vi "ManualClimb.vi"   [LabVIEW 2020]
uses:
  Robot Global Data.vi
  Swerve Global Variables.vi
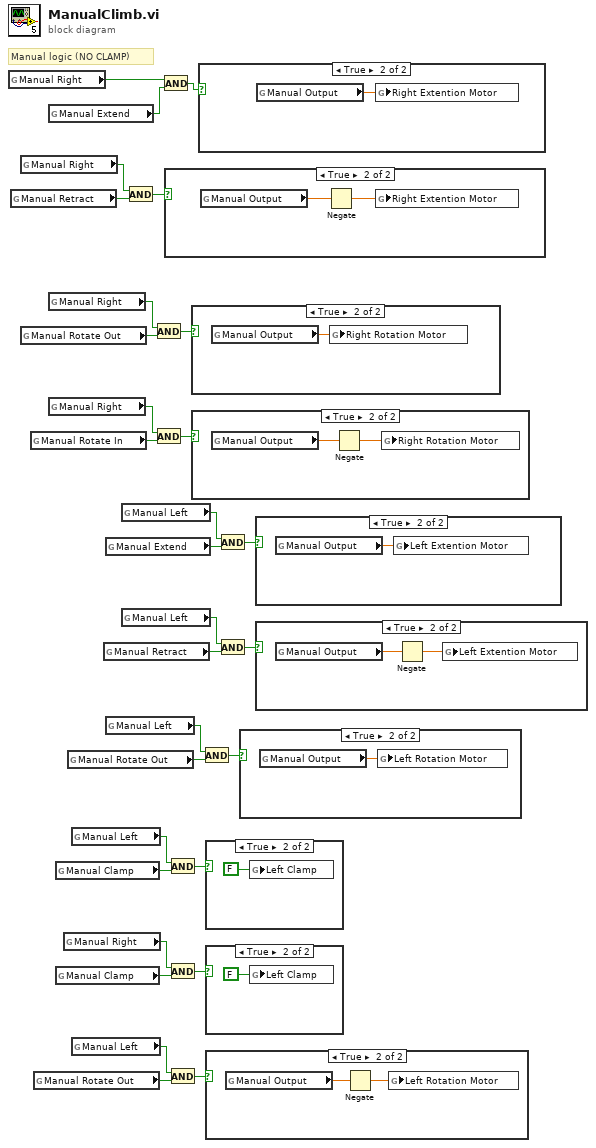
[diagram p0: block diagram]
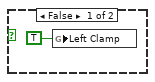
[diagram p2: hidden frame]
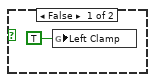
[diagram p3: hidden frame]
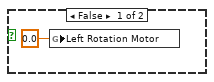
[diagram p4: hidden frame]
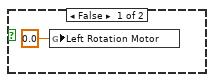
[diagram p5: hidden frame]
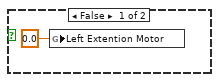
[diagram p6: hidden frame]
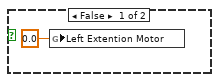
[diagram p7: hidden frame]
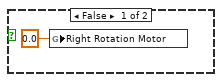
[diagram p8: hidden frame]
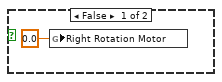
[diagram p9: hidden frame]
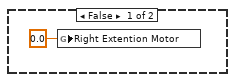
[diagram p10: hidden frame]
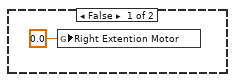
[diagram p11: hidden frame]
diagram:
  # "Manual logic (NO CLAMP)"
  n1 = global read "Robot Global Data.vi" "Manual Right"() -> (w2:bool)
  n2 = global read "Robot Global Data.vi" "Manual Retract"() -> (w5:bool)
  n3 = global read "Robot Global Data.vi" "Manual Right"() -> (w4:bool)
  n4 = global read "Robot Global Data.vi" "Manual Rotate Out"() -> (w9:bool)
  n5 = global read "Robot Global Data.vi" "Manual Rotate In"() -> (w12:bool)
  n6 = global read "Robot Global Data.vi" "Manual Rotate Out"() -> (w24:bool)
  n7 = global read "Robot Global Data.vi" "Manual Extend"() -> (w1:bool)
  n8 = global read "Robot Global Data.vi" "Manual Right"() -> (w8:bool)
  n9 = global read "Robot Global Data.vi" "Manual Right"() -> (w11:bool)
  n10 = global read "Robot Global Data.vi" "Manual Clamp"() -> (w26:bool)
  n11 = global read "Robot Global Data.vi" "Manual Clamp"() -> (w28:bool)
  n12 = global read "Robot Global Data.vi" "Manual Right"() -> (w27:bool)
  n13 = global read "Robot Global Data.vi" "Manual Rotate Out"() -> (w21:bool)
  n14 = global read "Robot Global Data.vi" "Manual Left"() -> (w25:bool)
  n15 = global read "Robot Global Data.vi" "Manual Left"() -> (w23:bool)
  n16 = global read "Robot Global Data.vi" "Manual Retract"() -> (w17:bool)
  n17 = global read "Robot Global Data.vi" "Manual Extend"() -> (w13:bool)
  n18 = global read "Robot Global Data.vi" "Manual Left"() -> (w20:bool)
  n19 = global read "Robot Global Data.vi" "Manual Left"() -> (w14:bool)
  n20 = global read "Robot Global Data.vi" "Manual Left"() -> (w16:bool)
  n21 = And(x=w4, y=w5) -> (x .and. y?=w6:bool)
  n22 = And(x=w8, y=w9) -> (x .and. y?=w7:bool)
  n23 = And(x=w11, y=w12) -> (x .and. y?=w10:bool)
  n24 = And(x=w2, y=w1) -> (x .and. y?=w3:bool)
  n25 = case shown="True" w6 {
    frame False {
      n26 = global write "Swerve Global Variables.vi" "Right Extention Motor"(0.0 ("Right Rotation Motor")) -> ()
    }
    frame True {
      n27 = global read "Swerve Global Variables.vi" "Manual Output"() -> (w33:dbl)
      n28 = Negate(x=w33) -> (-x=w32:dbl)
      n29 = global write "Swerve Global Variables.vi" "Right Extention Motor"(w32) -> ()
    }
  }
  n30 = And(x=w25, y=w26) -> (x .and. y?=w30:bool)
  n31 = And(x=w27, y=w28) -> (x .and. y?=w29:bool)
  n32 = And(x=w23, y=w24) -> (x .and. y?=w22:bool)
  n33 = case shown="True" w7 {
    frame False {
      n34 = global write "Swerve Global Variables.vi" "Right Rotation Motor"(0.0 ("Right Extention Motor")) -> ()
    }
    frame True {
      n35 = global read "Swerve Global Variables.vi" "Manual Output"() -> (w35:dbl)
      n36 = global write "Swerve Global Variables.vi" "Right Rotation Motor"(w35) -> ()
    }
  }
  n37 = case shown="True" w10 {
    frame False {
      n38 = global write "Swerve Global Variables.vi" "Right Rotation Motor"(0.0 ("Right Extention Motor")) -> ()
    }
    frame True {
      n39 = global read "Swerve Global Variables.vi" "Manual Output"() -> (w38:dbl)
      n40 = Negate(x=w38) -> (-x=w37:dbl)
      n41 = global write "Swerve Global Variables.vi" "Right Rotation Motor"(w37) -> ()
    }
  }
  n42 = case shown="True" w3 {
    frame False {
      n43 = global write "Swerve Global Variables.vi" "Right Extention Motor"(0.0 ("Right Rotation Motor")) -> ()
    }
    frame True {
      n44 = global read "Swerve Global Variables.vi" "Manual Output"() -> (w40:dbl)
      n45 = global write "Swerve Global Variables.vi" "Right Extention Motor"(w40) -> ()
    }
  }
  n46 = And(x=w20, y=w21) -> (x .and. y?=w19:bool)
  n47 = case shown="True" w30 {
    frame False {
      n48 = global write "Robot Global Data.vi" "Left Clamp"(TRUE ("Left Clamp")) -> ()
    }
    frame True {
      n49 = global write "Robot Global Data.vi" "Left Clamp"(FALSE ("Left Clamp")) -> ()
    }
  }
  n50 = case shown="True" w29 {
    frame False {
      n51 = global write "Robot Global Data.vi" "Left Clamp"(TRUE ("Left Clamp")) -> ()
    }
    frame True {
      n52 = global write "Robot Global Data.vi" "Left Clamp"(FALSE ("Left Clamp")) -> ()
    }
  }
  n53 = case shown="True" w22 {
    frame False {
      n54 = global write "Swerve Global Variables.vi" "Left Rotation Motor"(0.0 ("Left Rotation Motor")) -> ()
    }
    frame True {
      n55 = global read "Swerve Global Variables.vi" "Manual Output"() -> (w46:dbl)
      n56 = Negate(x=w46) -> (-x=w47:dbl)
      n57 = global write "Swerve Global Variables.vi" "Left Rotation Motor"(w47) -> ()
    }
  }
  n58 = And(x=w14, y=w13) -> (x .and. y?=w15:bool)
  n59 = And(x=w16, y=w17) -> (x .and. y?=w18:bool)
  n60 = case shown="True" w19 {
    frame False {
      n61 = global write "Swerve Global Variables.vi" "Left Rotation Motor"(0.0 ("Left Rotation Motor")) -> ()
    }
    frame True {
      n62 = global read "Swerve Global Variables.vi" "Manual Output"() -> (w49:dbl)
      n63 = global write "Swerve Global Variables.vi" "Left Rotation Motor"(w49) -> ()
    }
  }
  n64 = case shown="True" w15 {
    frame False {
      n65 = global write "Swerve Global Variables.vi" "Left Extention Motor"(0.0 ("Left Extention Motor")) -> ()
    }
    frame True {
      n66 = global read "Swerve Global Variables.vi" "Manual Output"() -> (w51:dbl)
      n67 = global write "Swerve Global Variables.vi" "Left Extention Motor"(w51) -> ()
    }
  }
  n68 = case shown="True" w18 {
    frame False {
      n69 = global write "Swerve Global Variables.vi" "Left Extention Motor"(0.0 ("Left Extention Motor")) -> ()
    }
    frame True {
      n70 = global read "Swerve Global Variables.vi" "Manual Output"() -> (w54:dbl)
      n71 = Negate(x=w54) -> (-x=w53:dbl)
      n72 = global write "Swerve Global Variables.vi" "Left Extention Motor"(w53) -> ()
    }
  }
